vi "Keithley 3330 Read.vi"(2 "Point #":i32, 3 "Instrument Address":refnum<visa-resource-name>) -> (0 "Stop":bool, 1 "Measurement":dbl[](array[numeric]) format="%.2e")   [LabVIEW 2024]
doc: "This VI reads a single reading from a Keithley 2001 multimeter. The stop boolean is always false. If no reading is obtained a single zero is returned.\nScott Hannahs, NHMFL-FSU, Nov 1993"
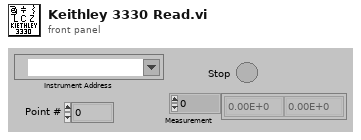
[diagram p1: front panel]
types:
  T1 = cluster{"Instrument":string, "ID Test String":string, "Terminator Character":string, u32, bool}
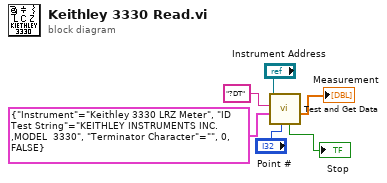
[diagram p0: block diagram]
diagram:
  n1 = call "Test and Get Data.vi"("Point #"="Point #", "Instrument Info"=T1 {"Instrument"="Keithley 3330 LRZ Meter", "ID Test String"="KEITHLEY INSTRUMENTS INC.,MODEL  3330", "Terminator Character"="", 0, FALSE}, "Command String"="?DT", "VISA Sesson"="Instrument Address") -> ("Measurement"=→"Measurement":dbl[], "Stop"=→"Stop":bool)  [unwired: 2 in, 3 out]
